vi "Save As Bmp.vi"(7 "ymax":i32, 9 "ymin":i32, 10 "palette":string, 11 "path":string) -> (1 "function return":u32, 2 "palette out":string, 3 "path out":string)   [LabVIEW 2018, in "AndorSDK.lvlib"]
doc: "EXPNETTYPE unsigned int WINAPI SaveAsBmp(char * path, char * palette, long ymin, long ymax);"
uses:
  AndorSDK.lvlib
  ATMCD32D.dll
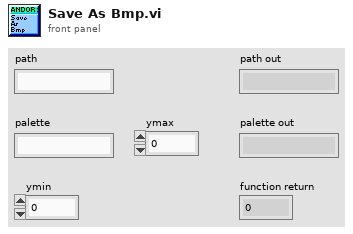
[diagram p1: front panel]
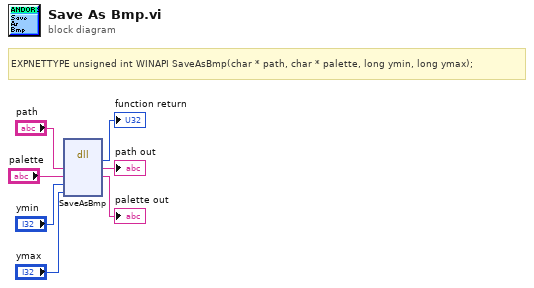
[diagram p0: block diagram]
diagram:
  # "EXPNETTYPE unsigned int WINAPI SaveAsBmp(char * path, char * palette, long ymin, long ymax);"
  n1 = dll-call lib="PTH2babs E\nPersönliches02 - Arbeit03-HiwijobsLabviewCodelibANDOR\tAndor SDK\nATMCD32D.*" fn="SaveAsBmp"("path"="path", "palette"="palette", "ymin"="ymin", "ymax"="ymax") -> (→"function return":u32, "path"=→"path out":string, "palette"=→"palette out":string)  [unwired: 5 in, 2 out]
